vi "EstimateAbsoluteOrientation3D.vi"(5 "Point Set Weights (Default: Empty - Equal Weights)":dbl[](array[numeric]), 7 "Epsilon (Default 1E-12)":dbl=1e-12 format="%#_13g", 8 "error in":errorcluster, 10 "Reference Point Set (Default - Use First  Set of Corresponding Points Array)":map{i32, T1}(c390), 11 "Object Point Sets":map{i32, T1}[](array[numeric])) -> (0 "error out":errorcluster, 1 "T Vectors":T1[](array[typedef]), 2 "R Matricies":dbl[][][](array[numeric]), 3 "Optimized Points":map{i32, T1}(c390), 4 "Scale Values":dbl[](array[numeric]))   [LabVIEW 2020, in "g_ar_toolkit.pointset_utils.lvlib"]
uses:
  g_ar_toolkit.pointset_utils.lvlib
  g_ar_toolkit.common/Object Point (Float).ctl
  bb6f7cf9-51dd-409a-b00a-fad66a2b610a.vi
  bb6f7cf9-51dd-409a-b00a-fad66a2b610a.vi/b761b6b4-53cc-4592-85b1-23315e9e6a73.vi
  Absolute Orientation/Absolute Orientation.lvlib
  g_ar_toolkit.common/g_ar_toolkit.common.lvlib
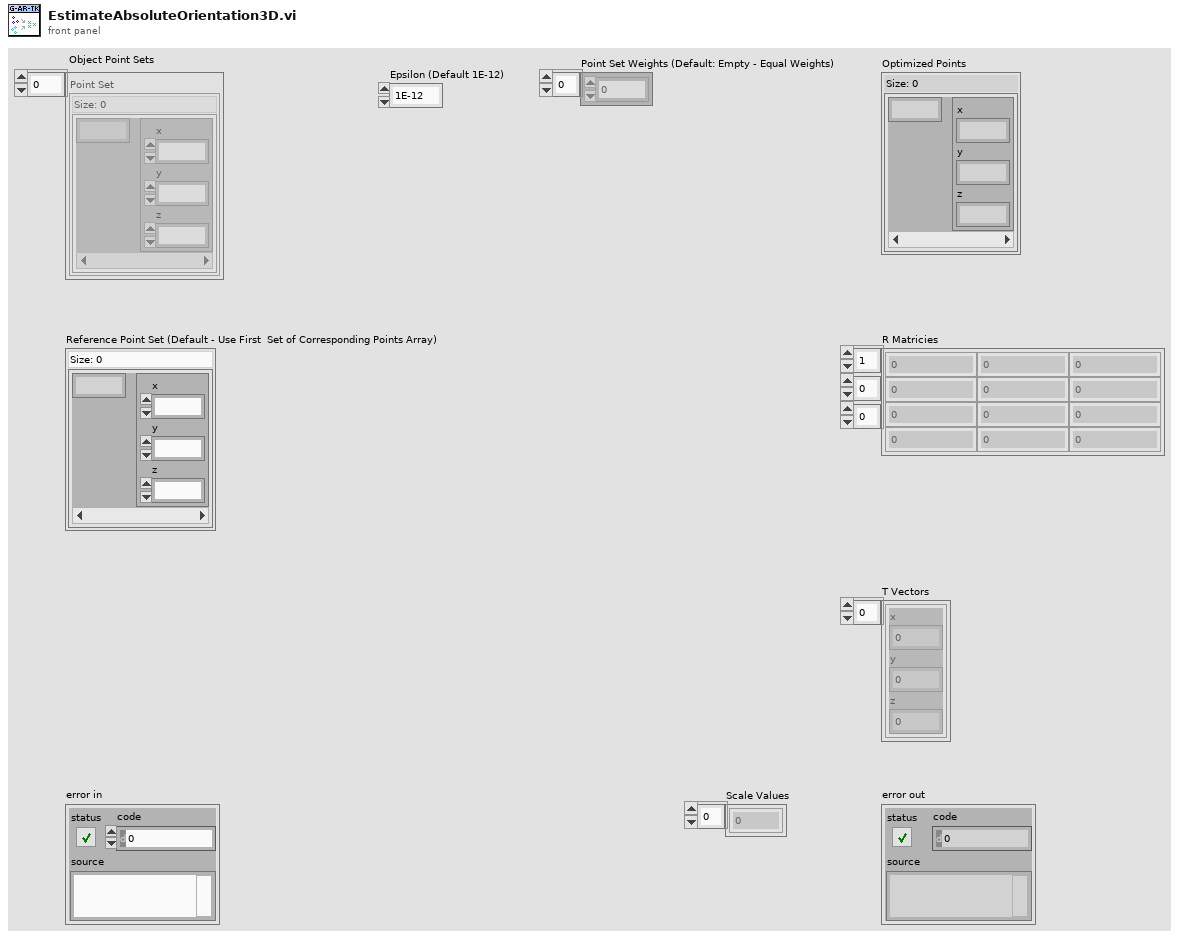
[diagram p1: front panel]
types:
  T1 = typedef "g_ar_toolkit.common.lvlib/Object Point (Float).ctl" = cluster{"x":dbl, "y":dbl, "z":dbl}
  T2 = typedef "g_ar_toolkit.pointset_utils.lvlib/Affine Estimation.lvlib/PointSet.ctl" = dbl[][]
  T3 = cluster{"T Vectors[0]":dbl, "T Vectors[1]":dbl, "T Vectors[2]":dbl}
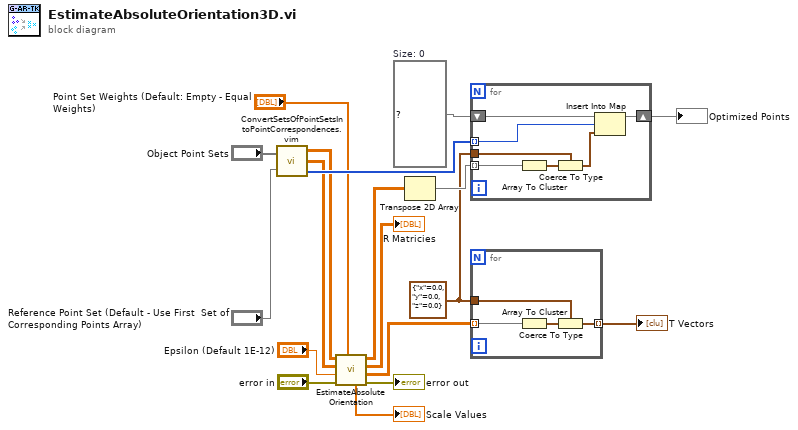
[diagram p0: block diagram]
diagram:
  w9 = map{i32, T1} {}  # Size: 0
  w4 = T1 {"x"=0.0, "y"=0.0, "z"=0.0} ("Point")
  n1 = call "ConvertSetsOfPointSetsIntoPointCorrespondences.vim"("Image Point Sets"="Object Point Sets", "Reference Point Set"="Reference Point Set (Default - Use First  Set of Corresponding Points Array)") -> ("Coresponding Point Sets"=w6:dbl[][][], "Reference Points"=w7:dbl[][], "Indicies"=w8:i32[])  [unwired: 1 in]
  n2 = call "EstimateAbsoluteOrientation.vi"("Point Set Weights"="Point Set Weights (Default: Empty - Equal Weights)", "error in"="error in", "Epsilon"="Epsilon (Default 1E-12)", "Reference Object Point"=w7, "Corresponding Object Points Array"=w6) -> ("error out"=→"error out":errorcluster, "T Vectors"=w3:dbl[][], "R Matricies"=→"R Matricies":dbl[][][], "Optimized Point Set"=w2:T2, "Scale Values"=→"Scale Values":dbl[])  [unwired: 2 in]
  n3 = Transpose 2D Array(2D array=w2) -> (transposed array=w5:T2)
  n4 = for {
    tunnel: w5 -> [w25] mode=indexing
    tunnel: w4 -> [w23]
    tunnel: w8 -> [w22] mode=indexing
    shift-right: [w20] -> w10
    shift-left: w9 -> [w19]
    n5 = Array To Cluster(array=w25) -> (cluster=w24:cluster{"[0]":dbl, "[1]":dbl, "[2]":dbl})
    n6 = Coerce To Type(0:w24, 1:w23) -> (2:w21:T1)
    n7 = Insert Into Map(map in=w19, key=w22, value=w21) -> (map out=w20:map{i32, T1})  [unwired: 2 out]
  }
  "Optimized Points" <- w10
  n8 = for {
    tunnel: w3 -> [w29] mode=indexing
    tunnel: w4 -> [w27]
    tunnel: [w26] -> w15 mode=indexing
    n9 = Array To Cluster(array=w29) -> (cluster=w28:T3)
    n10 = Coerce To Type(0:w28, 1:w27) -> (2:w26:T1)
  }
  "T Vectors" <- w15
